vi "test--load scheme and palette.vi"() -> ()   [LabVIEW 2021]
doc: "test the palette and scheme to see that things are getting loaded correctly\n\n--><b>Note:</b> Open the view VIs to see the color loading to verify\n\n<b>Code Developed By:</b>\nTechnology Service Corporation\n1983 S Liberty Drive\nBloomington, IN 47403\n\nDeveloper:\nDaniel Coons"
uses:
  Material Theme/Material Theme.lvclass
  Material-Scheme/Material-Scheme.lvclass
  Material-Palette/Material-Palette.lvclass
panel:
  in  "Theme":u16(ring)=3 items=["Light Theme", "Light Medium Contrast", "Light High Contrast", "Dark Theme", "Dark Medium Contrast", "Dark High Constrast"]
  in  "file path (use dialog)":path=path "C:/Users/daniel.coons/Downloads/mju-theme.xml"
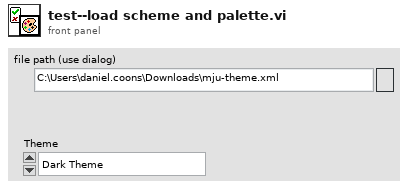
[diagram p1: front panel]
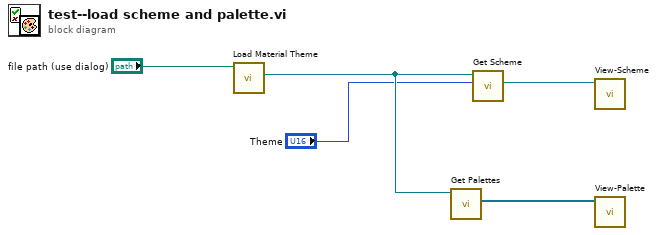
[diagram p0: block diagram]
diagram:
  n1 = call "Load Material Theme.vi"("file path (use dialog)"="file path (use dialog)") -> ("Theme"=w2:refnum<class "Material Theme.lvclass">)  [unwired: 9 in, 1 out]
  n2 = call "Get Palettes.vi"("Material Theme in"=w2) -> ("Material-Scheme"=w3:refnum<class "Material-Palette.lvclass">[])  [unwired: 8 in, 2 out]
  n3 = call "Get Scheme.vi"("Theme"="Theme", "Material Theme in"=w2) -> ("Material-Scheme"=w4:refnum<class "Material-Scheme.lvclass">)  [unwired: 7 in, 2 out]
  n4 = call "View-Scheme.vi"("Material-Scheme.lvclass"=w4) -> ()  [unwired: 11 in]
  n5 = call "View-Palette.vi"("Array"=w3) -> ()  [unwired: 11 in]
